vi "Actor Core.vi"(8 "error in":errorcluster, 11 "GUI View Actor in":refnum<class "GUI View Actor.lvclass">) -> (0 "error out":errorcluster, 3 "Actor out":refnum<class "Actor.lvclass">)   [LabVIEW 2017, in "GUI Views.lvlib" / "GUI View Actor.lvclass"]
doc: "(<B>Filename</B>: Actor Framework.lvlib:Actor.lvclass:Actor Core.vi)\n\nReceives messages to the actor, reacts to them, and initiates any error handling that may shut the actor down.\n\nDescendant classes may override this VI to append parallel tasks for the actor to complete while it handles messages. Overrides use the Call Parent Method node."
uses:
  GUI View Actor.lvclass
  <vilib>/ActorFramework/Actor/Actor.lvclass
  View Actor/View Actor.lvclass
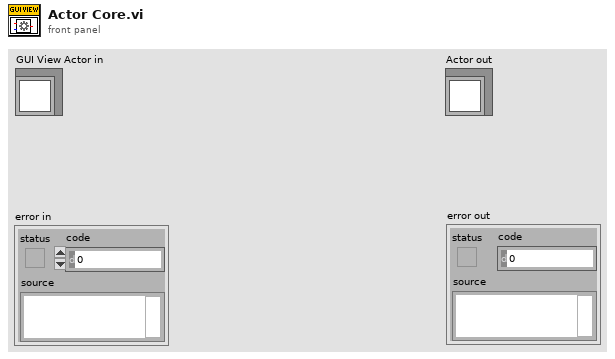
[diagram p1: front panel]
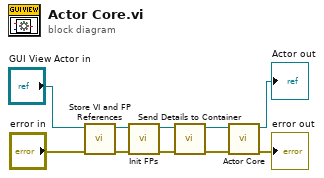
[diagram p0: block diagram]
diagram:
  n1 = call "Store VI and FP References.vi"("error in (no error)"="error in", "GUI View Actor in"="GUI View Actor in") -> ("error out"=w3:errorcluster, "GUI View Actor out"=w4:refnum<class "GUI View Actor.lvclass">)  [unwired: 8 in]
  n2 = call-dynamic "Init FPs.vi"("error in (no error)"=w3, "GUI View Actor in"=w4) -> ("error out"=w2:errorcluster, "GUI View Actor out"=w1:refnum<class "GUI View Actor.lvclass">)  [unwired: 8 in]
  n3 = call "Send Details to Container.vi"("error in (no error)"=w2, "GUI View Actor in"=w1) -> ("error out"=w6:errorcluster, "GUI View Actor out"=w5:refnum<class "GUI View Actor.lvclass">)  [unwired: 8 in]
  n4 = call-parent "Actor Core.vi"("error in"=w6, "Actor in"=w5) -> ("error out"=→"error out":errorcluster, "Actor out"=→"Actor out":refnum<class "Actor.lvclass">)  [unwired: 8 in]
